vi "Actor Core.vi"(8 "error in":errorcluster, 11 "Alpha UI in":refnum<class "Vehicle Position Interface Simulation.lvclass">) -> (0 "error out":errorcluster, 3 "Actor out":refnum<class "Actor.lvclass">)   [LabVIEW 2012, in "Vehical Position Interface Simulation.lvlib" / "Vehicle Position Interface Simulation.lvclass"]
doc: "(<B>Filename</B>: Actor Framework.lvlib:Actor.lvclass:Actor Core.vi)\n\nReceives messages to the actor, reacts to them, and initiates any error handling that may shut the actor down.\n\nDescendant classes may override this VI to append parallel tasks for the actor to complete while it handles messages. Overrides use the Call Parent Method node."
uses:
  Vehicle Position Interface Simulation.lvclass
  <vilib>/ActorFramework/Actor/Actor.lvclass
  <vilib>/ActorFramework/Stop Msg/Stop Msg.lvclass
  Vehical Position Interface API/Vehical Position Interface API/Vehicle Position Interface API.lvclass
  Car Wash Controller/Car Wash Controller/Car Wash Controller.lvclass
panel:
  in  "Vehicle Position Simulation":u8(slide) scale=0.0..4.0
  # "ENTRY"
  # "STATION 1"
  # "STATION 2"
  # "STATION 3"
  # "EXIT"
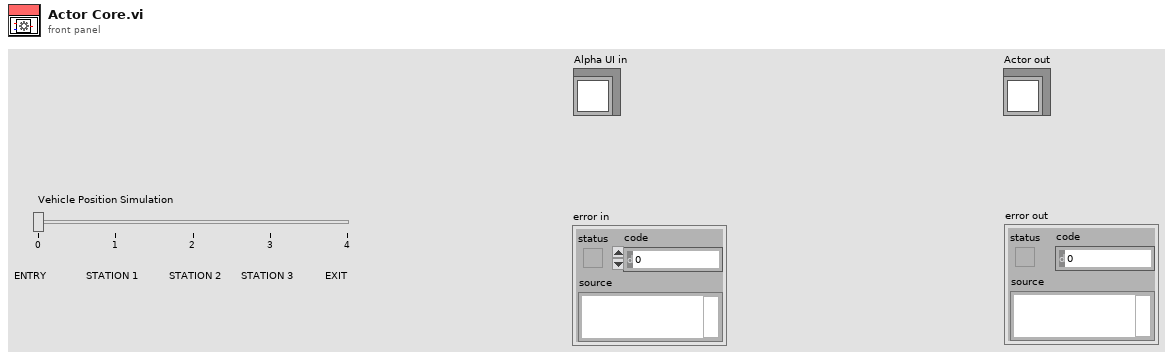
[diagram p1: front panel]
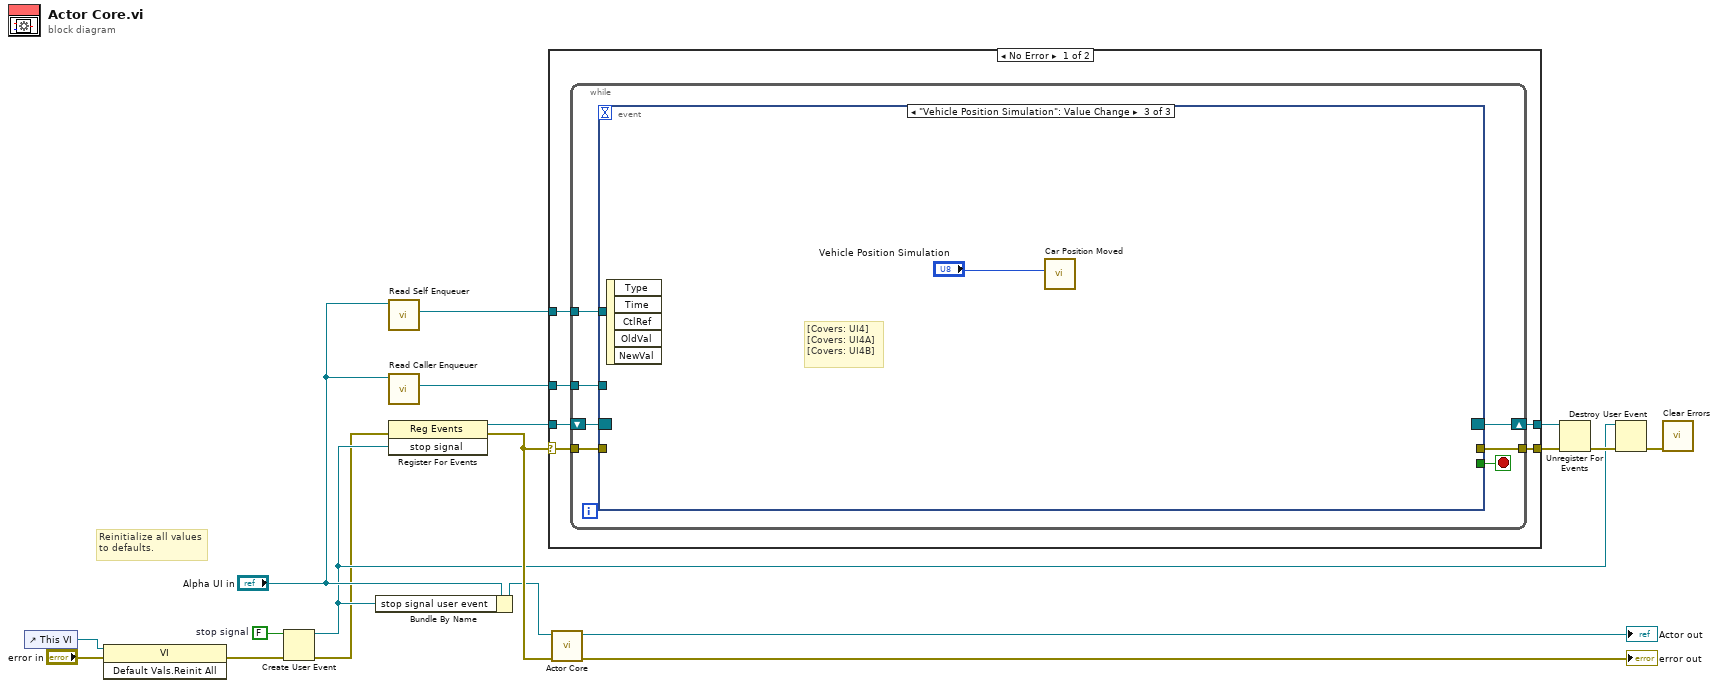
[diagram p0: block diagram]
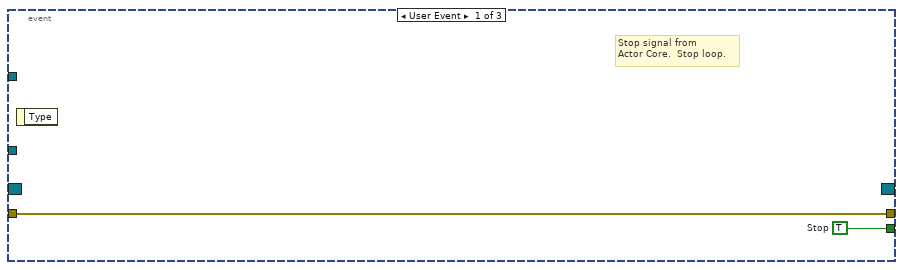
[diagram p2: hidden frame]
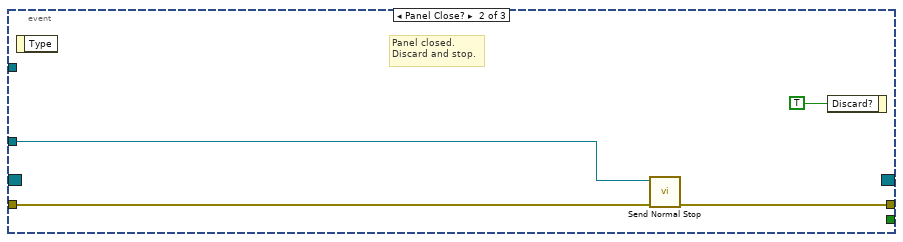
[diagram p3: hidden frame]
diagram:
  w16 = FALSE  # stop signal
  # "Reinitialize all values\nto defaults."
  n1 = control-ref of="This VI"() -> (w6:refnum<vi>)
  n2 = invoke class="VI" method="Default Vals.Reinit All"(reference=w6, error in="error in") -> (error out=w4:errorcluster)  [unwired: 1 in, 2 out]
  n3 = Create User Event(user event datatype=w16, error in=w4) -> (user event=w7:refnum<user-event>, error out=w3:errorcluster)
  n4 = Bundle By Name(cluster="Alpha UI in", "stop signal user event"=w7) -> (w1:refnum<class "Vehicle Position Interface Simulation.lvclass">)
  n5 = call <vilib>:"Read Self Enqueuer.vi"("Actor"="Alpha UI in") -> ("Self Enqueuer"=w18:refnum<class "Message Enqueuer.lvclass">)  [unwired: 10 in]
  n6 = call <vilib>:"Read Caller Enqueuer.vi"("Actor"="Alpha UI in") -> ("Caller Enqueuer"=w17:refnum<class "Message Enqueuer.lvclass">)  [unwired: 10 in]
  n7 = register-events(error in=w3, w7) -> (reference out=w15:refnum<event-registration>, error out=w12:errorcluster)  [unwired: 1 in]
  n8 = case shown="No Error" w12 {
    selector: w12 -> [w19 w39]
    tunnel: w18 -> [w24 _]
    tunnel: w17 -> [w23 _]
    tunnel: w15 -> [w22 w40]
    tunnel: [w21 w40] -> w13
    tunnel: [w20 w39] -> w11
    frame No Error {
      n9 = while {
        tunnel: w24 -> [w30]
        tunnel: w23 -> [w29]
        shift-right: [w27] -> w21
        shift-left: w22 -> [w28]
        tunnel: [w26] -> w20
        tunnel: w19 -> [w25]
        stop <- w31 stop-if-true
        n10 = event shown="[2] \"Vehicle Position Simulation\": Value Change" {
          selector: w28 -> [_ _ _]
          dyn-events: [_ _ _] -> w27
          timeout: _ -> [_ _ _]
          tunnel: [w33 _ _] -> w31
          tunnel: w30 -> [_ _ _]
          tunnel: w29 -> [_ w37 _]
          tunnel: [w32 w36 _] -> w26
          tunnel: w25 -> [w32 w35 _]
          event User Event {
            w33 = TRUE  # Stop
            # "Stop signal from\nActor Core.  Stop loop."
            n11 = event-data() -> ()  [unwired: 1 in, 1 out]
          }
          event Panel Close? {
            # "Panel closed.\nDiscard and stop."
            n12 = event-data() -> ()  [unwired: 1 in, 1 out]
            n13 = call <vilib>:"Send Normal Stop.vi"("error in (no error)"=w35, "Message Enqueuer"=w37) -> ("error out"=w36:errorcluster)  [unwired: 9 in]
            n14 = event-data("Discard?"=TRUE) -> ()  [unwired: 1 in, 1 out]
          }
          event "Vehicle Position Simulation": Value Change {
            # "[Covers: UI4]\n[Covers: UI4A]\n[Covers: UI4B]"
            n15 = event-data() -> ()  [unwired: 1 in, 5 out]
            n16 = call "Car Position Moved.vi"("Vehicle Position"="Vehicle Position Simulation") -> ()  [unwired: 9 in, 2 out]
          }
        }
      }
    }
    frame Error {
    }
  }
  n17 = call-parent "Actor Core.vi"("error in"=w12, "Actor in"=w1) -> ("error out"=→"error out":errorcluster, "Actor out"=→"Actor out":refnum<class "Actor.lvclass">)  [unwired: 8 in]
  n18 = Unregister For Events(event registration refnum=w13, error in=w11) -> (error out=w14:errorcluster)
  n19 = Destroy User Event(user event=w7, error in=w14) -> (error out=w2:errorcluster)
  n20 = call <vilib>:"Clear Errors.vi"("error in (no error)"=w2) -> ()  [unwired: 6 in, 1 out]
